vi "20220124-main.vi"() -> ()   [LabVIEW 2019]
panel:
  out "Image Out":T1(plugin-control)
  in  "Stop (F)":bool=TRUE
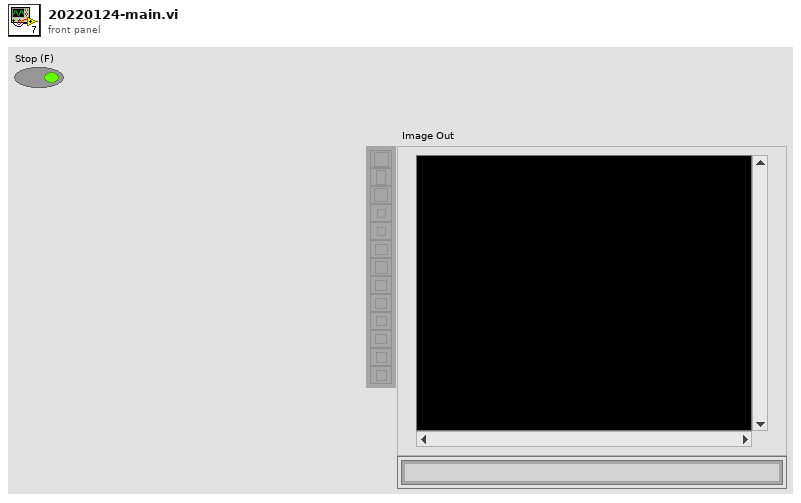
[diagram p1: front panel]
types:
  T1 = typedef "IMAQ Image.ctl" = refnum<image>
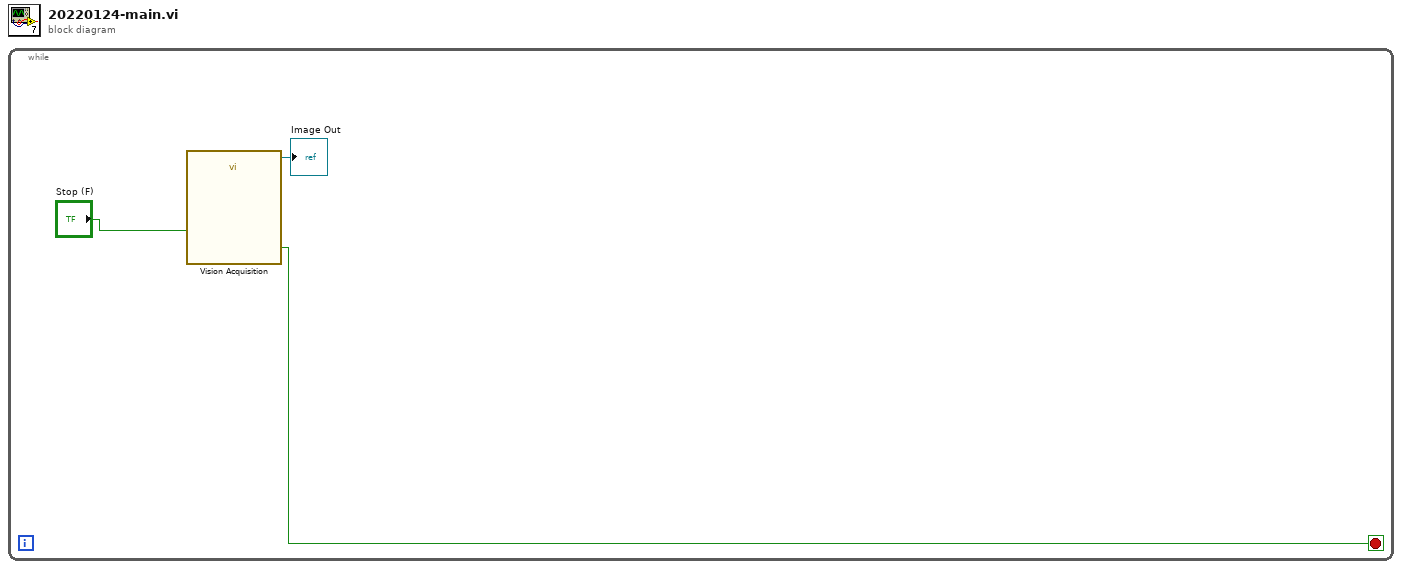
[diagram p0: block diagram]
diagram:
  n1 = while {
    stop <- w2 stop-if-true
    n2 = call "Vision Acquisition"("Stop (F)"="Stop (F)") -> ("Image Out"=→"Image Out":T1, "Stopped"=w2:bool)  [unwired: 24 in, 1 out]
  }
